vi "4-bit counter.vi"(0 "?":u16(ring) items=["up count", "down count"], 1 "clock (T/2) ms":u32, 2 "reset":bool) -> (3 "Q 4":bool=TRUE, 4 "Q 3":bool=TRUE, 5 "Q 2":bool=TRUE, 6 "Q":bool=TRUE)   [LabVIEW 2018]
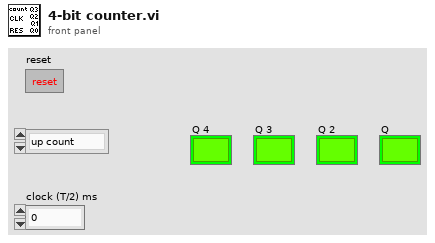
[diagram p1: front panel]
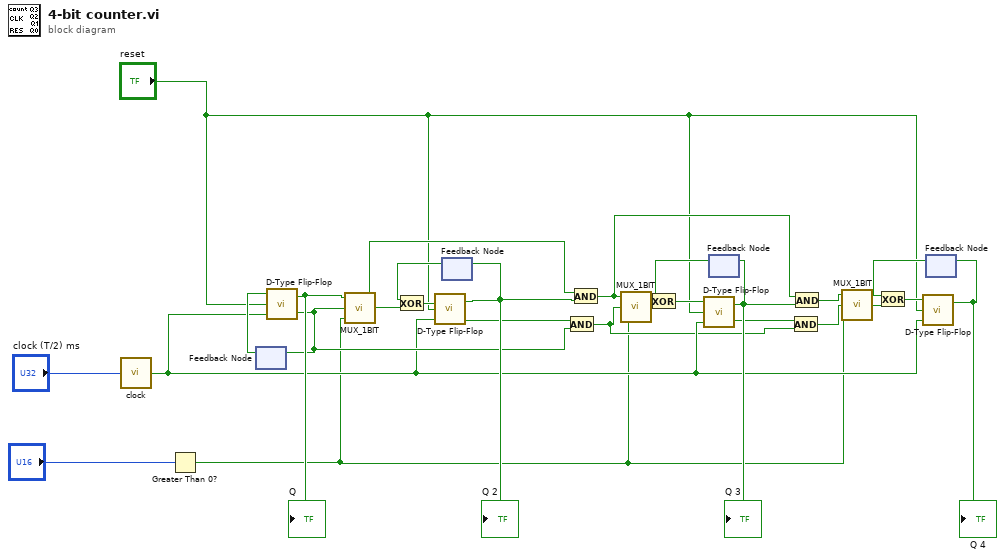
[diagram p0: block diagram]
diagram:
  n1 = call "clock.vi"("milliseconds to wait"="clock (T/2) ms") -> ("Q 2"=w8:bool)
  n2 = Greater Than 0?(x="?") -> (x > 0?=w1:bool)
  n3 = feedback #1() -> (w26:bool)  [unwired: 1 in]
  n4 = call "D-Type Flip-Flop.vi"("clock"=w8, "rest"="reset", "Data"=w26) -> ("!Q"=w16:bool, "Q"=w19:bool)
  "Q" <- w19
  n5 = feedback-in #1(w16) -> ()
  n6 = call "MUX_1BIT.vi"("S"=w1, "A2"=w16, "A1"=w19) -> ("Z"=w20:bool)
  n7 = feedback #2() -> (w24:bool)  [unwired: 1 in]
  n8 = Exclusive Or(1:w20, 2:w24) -> (0:w25:bool)
  n9 = call "D-Type Flip-Flop.vi"("clock"=w8, "rest"="reset", "Data"=w25) -> ("!Q"=w17:bool, "Q"=w23:bool)
  "Q 2" <- w23
  n10 = feedback-in #2(w23) -> ()
  n11 = And(x=w17, y=w16) -> (x .and. y?=w5:bool)
  n12 = And(x=w20, y=w23) -> (x .and. y?=w12:bool)
  n13 = call "MUX_1BIT.vi"("S"=w1, "A2"=w5, "A1"=w12) -> ("Z"=w18:bool)
  n14 = feedback #3() -> (w21:bool)  [unwired: 1 in]
  n15 = Exclusive Or(1:w18, 2:w21) -> (0:w22:bool)
  n16 = call "D-Type Flip-Flop.vi"("clock"=w8, "rest"="reset", "Data"=w22) -> ("!Q"=w6:bool, "Q"=w11:bool)
  "Q 3" <- w11
  n17 = feedback-in #3(w11) -> ()
  n18 = And(x=w6, y=w5) -> (x .and. y?=w2:bool)
  n19 = And(x=w12, y=w11) -> (x .and. y?=w3:bool)
  n20 = call "MUX_1BIT.vi"("S"=w1, "A2"=w2, "A1"=w3) -> ("Z"=w4:bool)
  n21 = feedback #4() -> (w10:bool)  [unwired: 1 in]
  n22 = Exclusive Or(1:w4, 2:w10) -> (0:w13:bool)
  n23 = call "D-Type Flip-Flop.vi"("clock"=w8, "rest"="reset", "Data"=w13) -> ("Q"=w7:bool)  [unwired: 1 out]
  "Q 4" <- w7
  n24 = feedback-in #4(w7) -> ()
